vi "Constants.vi"() -> ()   [LabVIEW 2023, in "AFPP Shared.lvlib"]
uses:
  AFPP Shared.lvlib
panel:
  in  "Actors":string="AMA.Actors"
  in  "Actor Paths":string="AMA.ActorPaths"
  in  "PPL Tag":string="AMA.PPL"
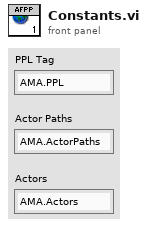
[diagram p1: front panel]
diagram:
